vi "Streame to Matlab.vi"(9 "Intensity":refnum<vi>, 10 "range":refnum<vi>, 11 "StopRef":refnum<vi>) -> ()   [LabVIEW 2013]
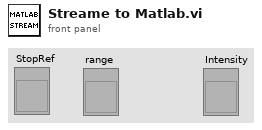
[diagram p1: front panel]
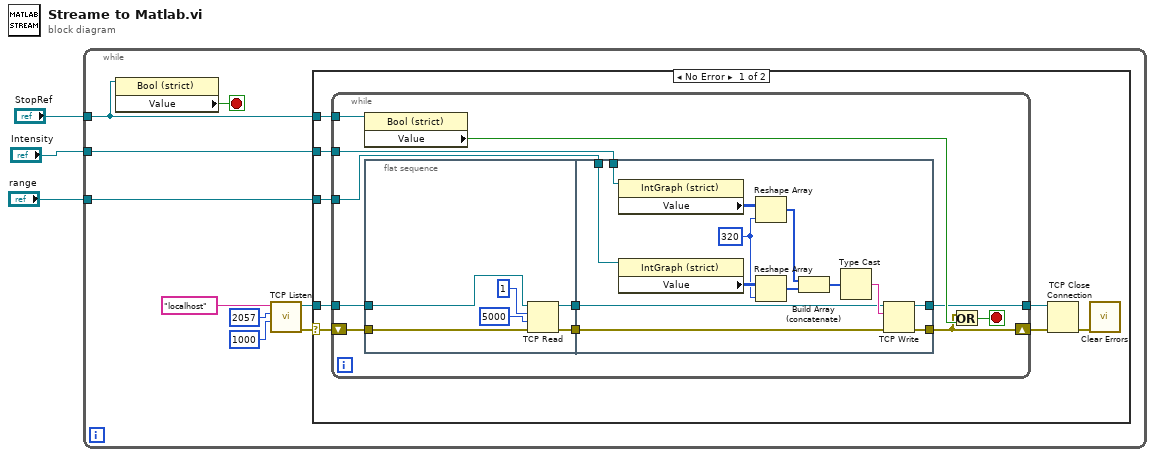
[diagram p0: block diagram]
diagram:
  n1 = while {
    tunnel: "StopRef" -> [w6]
    tunnel: "range" -> [w5]
    tunnel: "Intensity" -> [w4]
    stop <- w8 stop-if-true
    n2 = property class="Bool (strict)"(reference=w6) -> ("Value"=w8:bool)  [unwired: 1 in, 2 out]
    n3 = call <vilib>:"TCP Listen.vi"("timeout ms (wait forever: -1)"=1000, "port"=u16 2057, "service name"="localhost" ("address")) -> ("error out"=w7:errorcluster, "connection ID"=w12:refnum<k5>)  [unwired: 4 in, 3 out]
    n4 = case shown="No Error" w7 {
      selector: w7 -> [w16 _]
      tunnel: w12 -> [w18 _]
      tunnel: w6 -> [w15 _]
      tunnel: w5 -> [w14 _]
      tunnel: w4 -> [w13 _]
      frame No Error {
        n5 = while {
          tunnel: w18 -> [w31]
          tunnel: [w26] -> w19
          shift-right: [w24] -> w20
          shift-left: w16 -> [w30]
          tunnel: w15 -> [w23]
          tunnel: w14 -> [w22]
          tunnel: w13 -> [w21]
          stop <- w25 stop-if-true
          n6 = property class="Bool (strict)"(reference=w23) -> ("Value"=w29:bool)  [unwired: 1 in, 2 out]
          n7 = flat-sequence {
            tunnel: w31 -> [w34]
            tunnel: w30 -> [w33]
            tunnel: [w37] -> w28
            tunnel: [w36] -> w27
            tunnel: w28 -> [w48]
            tunnel: w27 -> [w47]
            tunnel: [w46] -> w26
            tunnel: [w45] -> w24
            tunnel: w22 -> [w39]
            tunnel: w21 -> [w38]
            frame #0 {
              n8 = TCP Read(connection ID=w34, bytes to read=1, error in (no error)=w33, 9:5000 ("timeout ms (25000)")) -> (connection ID out=w37:refnum<k5>, error out=w36:errorcluster)  [unwired: 1 in, 1 out]
            }
            frame #1 {
              w40 = 320 ("dimension size")
              n9 = property class="IntGraph (strict)"(reference=w38) -> ("Value"=w44:i32[][])  [unwired: 1 in, 2 out]
              n10 = property class="IntGraph (strict)"(reference=w39) -> ("Value"=w50:u32[][])  [unwired: 1 in, 2 out]
              n11 = Reshape Array(w44, w40) -> (w43:i32[])
              n12 = Reshape Array(w50, w40) -> (w42:u32[])
              n13 = Build Array (concatenate)(w43, w42) -> (w41:u32[])
              n14 = Type Cast(x=w41) -> (*(type *) &x=w49:string)  [unwired: 1 in]
              n15 = TCP Write(connection ID=w48, data in=w49, error in (no error)=w47) -> (connection ID out=w46:refnum<k5>, error out=w45:errorcluster)  [unwired: 1 in, 1 out]
            }
          }
          n16 = Or(x=w24, y=w29) -> (x .or. y?=w25:bool)
        }
        n17 = TCP Close Connection(connection ID=w19, error in (no error)=w20) -> (error out=w17:errorcluster)  [unwired: 1 in, 1 out]
        n18 = call <vilib>:"Clear Errors.vi"("error in (no error)"=w17) -> ()  [unwired: 6 in, 1 out]
      }
      frame Error {
      }
    }
  }
